vi "RSA Verify Hash.vi"(7 "public_key":string, 8 "error in (no error)":errorcluster, 9 "data":u8[](array[numeric]), 10 "signed_data":u8[](array[numeric]), 11 "RSA in":refnum<class "RSA.lvclass">) -> (0 "error out":errorcluster, 2 "verify?":bool, 3 "RSA out":refnum<class "RSA.lvclass">)   [LabVIEW 2023, in "RSA.lvclass"]
uses:
  RSA.lvclass
  RSA.lvclass/RSA.ctl
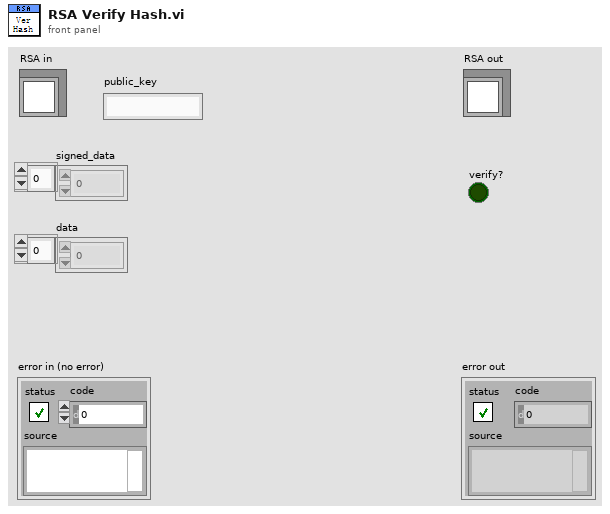
[diagram p1: front panel]
types:
  T1 = enum16{"MD5", "SHA1", "SHA256", "SHA384", "SHA512"}
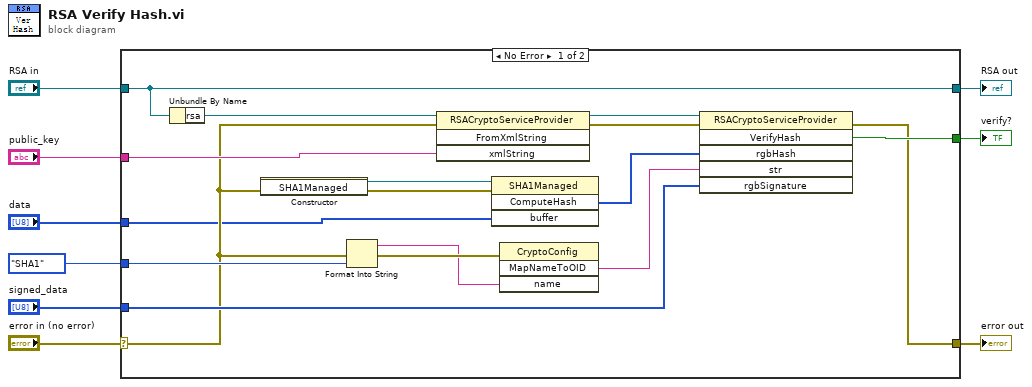
[diagram p0: block diagram]
diagram:
  n1 = case shown="No Error" "error in (no error)" {
    selector: "error in (no error)" -> [w11 w28]
    tunnel: [w12 w28] -> w8
    tunnel: [w26 w27] -> w6
    tunnel: "RSA in" -> [w26 w27]
    tunnel: [w22 _] -> w5
    tunnel: "public_key" -> [w21 _]
    tunnel: T1."SHA1" ("oid_type") -> [w14 _]
    tunnel: "signed_data" -> [w13 _]
    tunnel: "data" -> [w10 _]
    frame No Error {
      n2 = Unbundle By Name(w26) -> ("rsa"=w25:refnum<k24>)
      n3 = constructor class="SHA1Managed" ("AliceEntschlüsselt")(error in=w11) -> (reference out=w16:refnum<k24>, error out=w17:errorcluster)  [unwired: 2 in, 1 out]
      n4 = Format Into String(error in=w11, w14) -> (resulting string=w19:string, error out=w20:errorcluster)  [unwired: 2 in]
      n5 = invoke class="RSACryptoServiceProvider" method="FromXmlString"(reference=w25, error in=w11, "xmlString"=w21) -> (reference out=w23:refnum<k24>, error out=w24:errorcluster)  [unwired: 1 in, 2 out]
      n6 = invoke class="SHA1Managed" method="ComputeHash"(reference=w16, error in=w17, "buffer"=w10) -> ("ComputeHash"=w15:u8[])  [unwired: 1 in, 3 out]
      n7 = invoke class="CryptoConfig" method="MapNameToOID"(error in=w20, "name"=w19) -> ("MapNameToOID"=w18:string)  [unwired: 2 in, 3 out]
      n8 = invoke class="RSACryptoServiceProvider" method="VerifyHash"(reference=w23, error in=w24, "rgbHash"=w15, "str"=w18, "rgbSignature"=w13) -> (error out=w12:errorcluster, "VerifyHash"=w22:bool)  [unwired: 1 in, 4 out]
    }
    frame Error {
    }
  }
  "error out" <- w8
  "RSA out" <- w6
  "verify?" <- w5
